vi "MVC OOP Advanced.vi"() -> ()   [LabVIEW 2011]
doc: "This VI is a basic function generator utilising a class to encapsulate frequency type and the resultant waveform"
uses:
  Controls/Waveform Type.ctl
  Controls/Command.ctl
  Advanced Waveform Class/Advanced Waveform.lvclass
panel:
  in  "Waveform Type":T1
  in  "FFT Signal":bool
  in  "Gen Signal":bool
  in  "Frequency":dbl(knob) scale=0.0..11.0
  out "Waveform Graph":waveform(dbl)(graph)
  in  "stop":bool
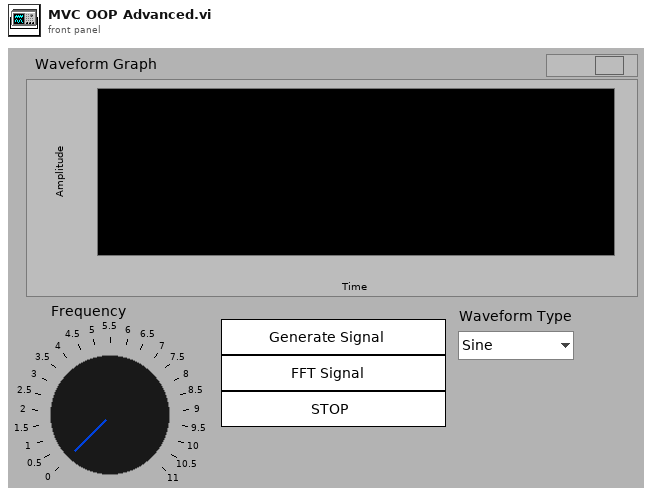
[diagram p1: front panel]
types:
  T1 = typedef "Waveform Type.ctl" = enum16{"Sine", "Square", "Triangle"}
  T2 = typedef "Command.ctl" = enum16{"Create Signal", "FFT Signal", "Set Frequency", "Stop", "Display", "Set Type"}
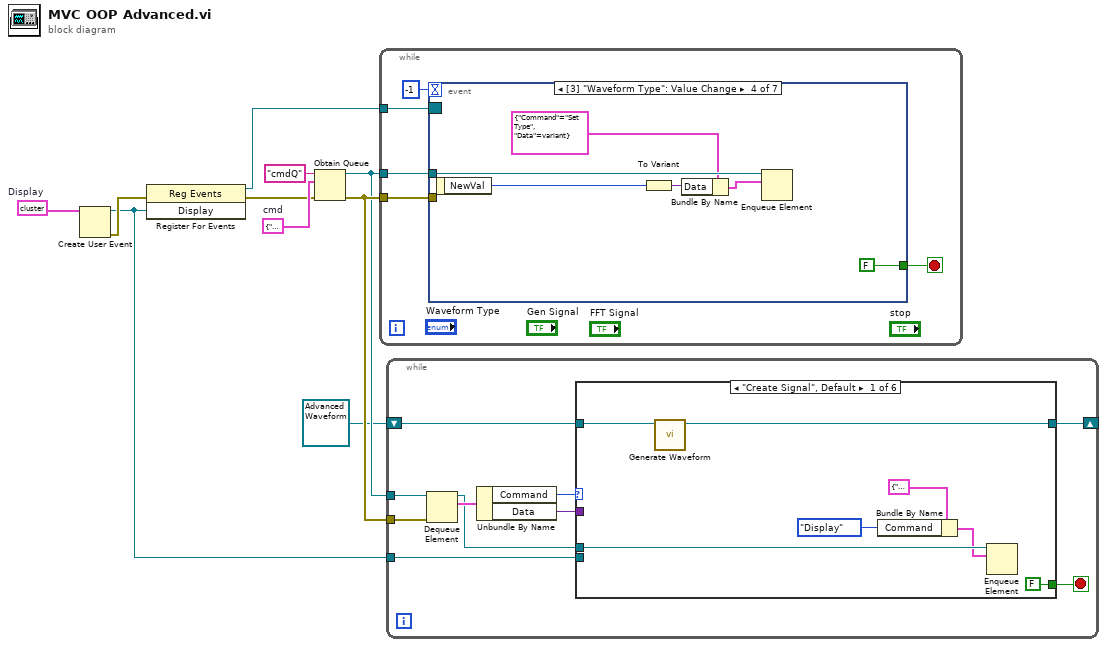
[diagram p0: block diagram]
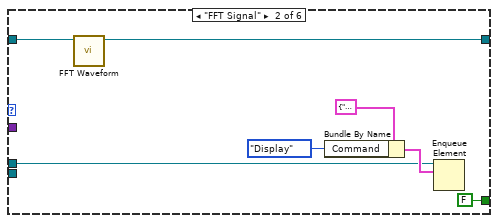
[diagram p2: hidden frame]
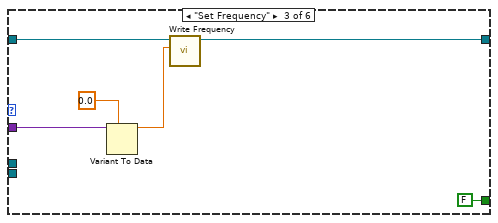
[diagram p3: hidden frame]
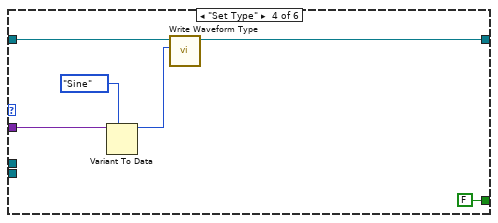
[diagram p4: hidden frame]
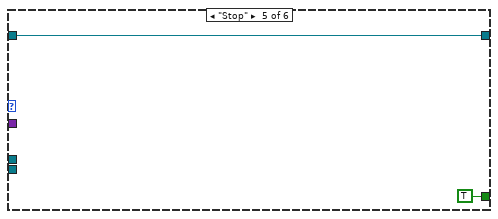
[diagram p5: hidden frame]
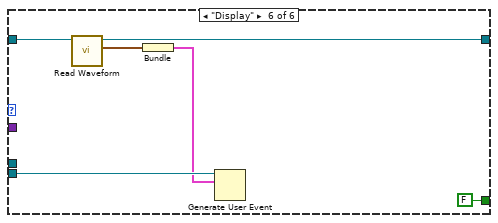
[diagram p6: hidden frame]
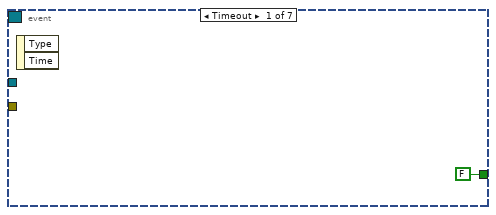
[diagram p7: hidden frame]
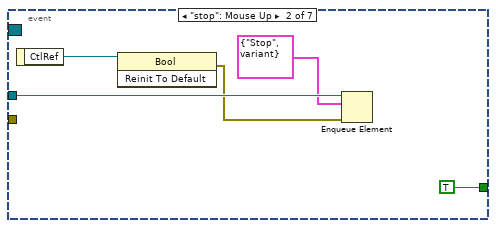
[diagram p8: hidden frame]
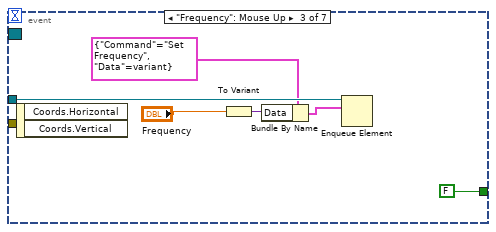
[diagram p9: hidden frame]
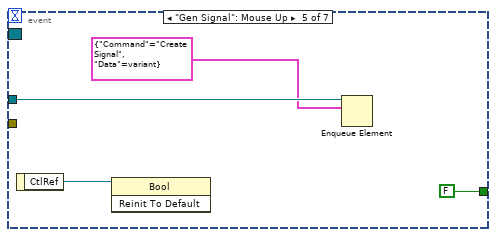
[diagram p10: hidden frame]
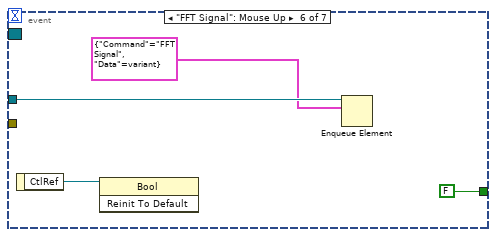
[diagram p11: hidden frame]
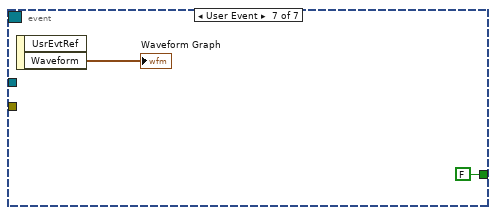
[diagram p12: hidden frame]
diagram:
  w7 = cluster{"Waveform":waveform(dbl)} {"Waveform"={"t0"=timestamp(0 s since 1904-01-01), "dt"=1.0, "Y"=[]}}  # Display
  w10 = cluster{"Command":T2, "Data":variant} {"Command"=enum."Create Signal", "Data"=variant}  # cmd
  n1 = Create User Event(user event datatype=w7) -> (user event=w2:refnum<user-event>, error out=w6:errorcluster)  [unwired: 1 in]
  n2 = register-events(error in=w6, w2) -> (reference out=w5:refnum<event-registration>, error out=w8:errorcluster)  [unwired: 1 in]
  n3 = Obtain Queue(name (unnamed)="cmdQ", element data type=w10, error in (no error)=w8) -> (queue out=w3:refnum<queue>, error out=w4:errorcluster)  [unwired: 2 in, 1 out]
  n4 = while {
    tunnel: w3 -> [w14]
    tunnel: w5 -> [w12]
    tunnel: w4 -> [w11]
    stop <- w13 stop-if-true
    n5 = event shown="[3] \"Waveform Type\": Value Change" {
      selector: w12 -> [_ _ _ _ _ _ _]
      dyn-events: _ -> [_ _ _ _ _ _ _]
      timeout: -1 -> [_ _ _ _ _ _ _]
      tunnel: w14 -> [_ w20 w27 w33 w37 w41 _]
      tunnel: [FALSE TRUE FALSE FALSE FALSE FALSE FALSE] -> w13
      tunnel: w11 -> [_ _ _ _ _ _ _]
      event Timeout {
        n6 = event-data() -> ()  [unwired: 1 in, 2 out]
      }
      event "stop": Mouse Up {
        n7 = event-data() -> ("CtlRef"=w21:refnum<vi>)  [unwired: 1 in]
        n8 = invoke class="Bool" method="Reinit To Default"(reference=w21) -> (error out=w19:errorcluster)  [unwired: 2 in, 2 out]
        n9 = Enqueue Element(queue=w20, element=cluster{"Command":T2, "Data":variant} {"Command"=enum."Stop", "Data"=variant}, error in (no error)=w19) -> ()  [unwired: 1 in, 3 out]
      }
      event "Frequency": Mouse Up {
        n10 = event-data() -> ()  [unwired: 1 in, 2 out]
        n11 = To Variant(anything="Frequency") -> (Variant=w23:variant)
        n12 = Bundle By Name(cluster=cluster{"Command":T2, "Data":variant} {"Command"=enum."Set Frequency", "Data"=variant} ("element"), "Data"=w23) -> (w24:cluster{"Command":T2, "Data":variant})
        n13 = Enqueue Element(queue=w27, element=w24) -> ()  [unwired: 2 in, 3 out]
      }
      event Value Change {
        n14 = event-data() -> ("NewVal"=w28:T1)  [unwired: 1 in]
        n15 = To Variant(anything=w28) -> (Variant=w29:variant)
        n16 = Bundle By Name(cluster=cluster{"Command":T2, "Data":variant} {"Command"=enum."Set Type", "Data"=variant} ("element"), "Data"=w29) -> (w30:cluster{"Command":T2, "Data":variant})
        n17 = Enqueue Element(queue=w33, element=w30) -> ()  [unwired: 2 in, 3 out]
      }
      event "Gen Signal": Mouse Up {
        n18 = event-data() -> ("CtlRef"=w34:refnum<vi>)  [unwired: 1 in]
        n19 = invoke class="Bool" method="Reinit To Default"(reference=w34) -> ()  [unwired: 2 in, 3 out]
        n20 = Enqueue Element(queue=w37, element=cluster{"Command":T2, "Data":variant} {"Command"=enum."Create Signal", "Data"=variant}) -> ()  [unwired: 2 in, 3 out]
      }
      event "FFT Signal": Mouse Up {
        n21 = event-data() -> ("CtlRef"=w38:refnum<vi>)  [unwired: 1 in]
        n22 = invoke class="Bool" method="Reinit To Default"(reference=w38) -> ()  [unwired: 2 in, 3 out]
        n23 = Enqueue Element(queue=w41, element=cluster{"Command":T2, "Data":variant} {"Command"=enum."FFT Signal", "Data"=variant}) -> ()  [unwired: 2 in, 3 out]
      }
      event User Event {
        n24 = event-data() -> ("Waveform"=→"Waveform Graph":waveform(dbl))  [unwired: 1 in, 1 out]
      }
    }
  }
  n25 = while {
    tunnel: w4 -> [w52]
    tunnel: w3 -> [w53]
    tunnel: w2 -> [w46]
    shift-right: [w44] -> _
    shift-left: refnum<class "Advanced Waveform.lvclass"> refnum ("Advanced Waveform.lvclass") -> [w45]
    stop <- w48 stop-if-true
    n26 = Dequeue Element(queue=w53, error in (no error)=w52) -> (queue out=w47:refnum<queue>, element=w51:cluster{"Command":T2, "Data":variant})  [unwired: 1 in, 2 out]
    n27 = Unbundle By Name(w51) -> ("Command"=w50:T2, "Data"=w49:variant)
    n28 = case shown="\"Create Signal\", Default" w50 {
      tunnel: w49 -> [_ _ w73 w79 _ _]
      tunnel: [FALSE FALSE FALSE FALSE TRUE FALSE] -> w48
      tunnel: w47 -> [w60 w64 _ _ _ _]
      tunnel: w46 -> [_ _ _ _ _ w87]
      tunnel: w45 -> [w55 w62 w71 w77 w80 w84]
      tunnel: [w54 w61 w68 w75 w80 w82] -> w44
      frame "Create Signal", Default {
        n29 = call-dynamic "Generate Waveform.vi"("Waveform in"=w55) -> ("Waveform out"=w54:refnum<class "Advanced Waveform.lvclass">)  [unwired: 9 in, 1 out]
        n30 = Bundle By Name(cluster=cluster{"Command":T2, "Data":variant} {"Command"=enum."Create Signal", "Data"=variant} ("element"), "Command"=Command."Display") -> (w57:cluster{"Command":T2, "Data":variant})
        n31 = Enqueue Element(queue=w60, element=w57) -> ()  [unwired: 2 in, 3 out]
      }
      frame "FFT Signal" {
        n32 = call-dynamic "FFT Waveform.vi"("Waveform in"=w62) -> ("Waveform out"=w61:refnum<class "Advanced Waveform.lvclass">)  [unwired: 9 in, 1 out]
        n33 = Bundle By Name(cluster=cluster{"Command":T2, "Data":variant} {"Command"=enum."Create Signal", "Data"=variant} ("element"), "Command"=Command."Display") -> (w65:cluster{"Command":T2, "Data":variant})
        n34 = Enqueue Element(queue=w64, element=w65) -> ()  [unwired: 2 in, 3 out]
      }
      frame "Set Frequency" {
        n35 = Variant To Data(type=0.0 ("Frequency"), Variant=w73) -> (data=w69:dbl)  [unwired: 1 in, 1 out]
        n36 = call-dynamic "Write Frequency.vi"("Frequency"=w69, "Waveform in"=w71) -> ("Waveform out"=w68:refnum<class "Advanced Waveform.lvclass">)  [unwired: 8 in, 1 out]
      }
      frame "Set Type" {
        n37 = Variant To Data(type=Waveform_Type."Sine" ("Waveform Type"), Variant=w79) -> (data=w76:T1)  [unwired: 1 in, 1 out]
        n38 = call-dynamic "Write Waveform Type.vi"("Waveform Type"=w76, "Advanced Waveform in"=w77) -> ("Advanced Waveform out"=w75:refnum<class "Advanced Waveform.lvclass">)  [unwired: 8 in, 1 out]
      }
      frame "Stop" {
      }
      frame "Display" {
        n39 = call-dynamic "Read Waveform.vi"("Waveform in"=w84) -> ("Waveform"=w83:waveform(dbl), "Waveform out"=w82:refnum<class "Advanced Waveform.lvclass">)  [unwired: 8 in, 1 out]
        n40 = Bundle("Waveform"=w83) -> (w86:cluster{"Waveform":waveform(dbl)})  [unwired: 1 in]
        n41 = Generate User Event(user event=w87, event data cluster=w86) -> ()  [unwired: 1 in, 2 out]
      }
    }
  }
